vi "Picture Ring Index from PID.vi"(1 "myRIO PID":string) -> (0 "picture ring index":u32)   [LabVIEW 2021]
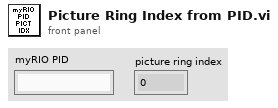
[diagram p1: front panel]
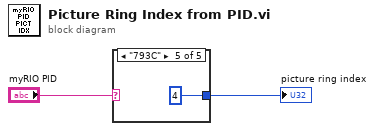
[diagram p0: block diagram]
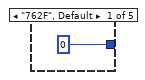
[diagram p2: hidden frame]
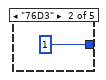
[diagram p3: hidden frame]
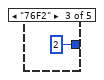
[diagram p4: hidden frame]
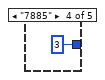
[diagram p5: hidden frame]
diagram:
  n1 = case shown="\"793C\"" "myRIO PID" {
    tunnel: [u32 0 u32 1 u32 2 u32 3 u32 4] -> w1
    frame "762F", Default {
    }
    frame "76D3" {
    }
    frame "76F2" {
    }
    frame "7885" {
    }
    frame "793C" {
    }
  }
  "picture ring index" <- w1
